vi "QuaternionDecode.vi"(8 "qw":dbl, 9 "qz":dbl, 10 "qy":dbl, 11 "qx":dbl) -> (1 "heading":dbl)   [LabVIEW 2009]
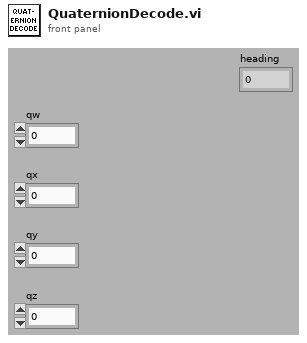
[diagram p1: front panel]
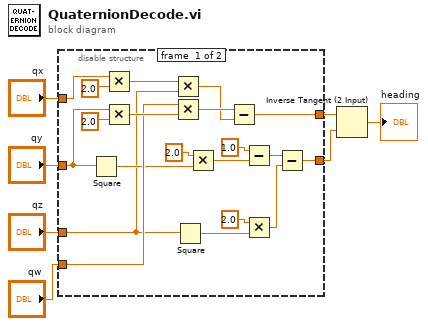
[diagram p0: block diagram]
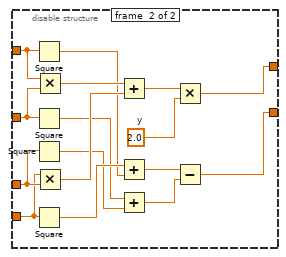
[diagram p2: hidden frame]
diagram:
  n1 = disable-structure shown="Enabled" {
    disable-tunnel: "qw" -> [w25 w36]
    disable-tunnel: "qx" -> [w23 w37]
    disable-tunnel: [w19 w29] -> w5
    disable-tunnel: "qy" -> [w17 w38]
    disable-tunnel: "qz" -> [w13 w39]
    disable-tunnel: [w8 w28] -> w2
    frame #0 {
      n2 = Square(x=w17) -> (x^2=w16:dbl)
      n3 = Multiply(x=w23, y=2.0) -> (x*y=w21:dbl)
      n4 = Multiply(x=w17, y=2.0) -> (x*y=w26:dbl)
      n5 = Multiply(x=w21, y=w13) -> (x*y=w20:dbl)
      n6 = Multiply(x=w25, y=w26) -> (x*y=w24:dbl)
      n7 = Square(x=w13) -> (x^2=w12:dbl)
      n8 = Multiply(x=2.0, y=w16) -> (x*y=w14:dbl)
      n9 = Subtract(x=w24, y=w20) -> (x-y=w19:dbl)
      n10 = Subtract(x=1.0, y=w14) -> (x-y=w10:dbl)
      n11 = Multiply(x=2.0, y=w12) -> (x*y=w9:dbl)
      n12 = Subtract(x=w10, y=w9) -> (x-y=w8:dbl)
    }
    frame #1 {
      w40 = 2.0  # y
      n13 = Square(x=w37) -> (x^2=w31:dbl)
      n14 = Square(x=w38) -> (x^2=w34:dbl)
      n15 = Square(x=w39) -> (x^2=w30:dbl)
      n16 = Square(x=w36) -> (x^2=w35:dbl)
      n17 = Multiply(x=w37, y=w38) -> (x*y=w43:dbl)
      n18 = Multiply(x=w36, y=w39) -> (x*y=w42:dbl)
      n19 = Add(x=w43, y=w42) -> (x+y=w41:dbl)
      n20 = Add(x=w35, y=w31) -> (x+y=w32:dbl)
      n21 = Add(x=w34, y=w30) -> (x+y=w33:dbl)
      n22 = Multiply(x=w41, y=w40) -> (x*y=w29:dbl)
      n23 = Subtract(x=w32, y=w33) -> (x-y=w28:dbl)
    }
  }
  n24 = Inverse Tangent (2 Input)(1:w2, 2:w5) -> (0:→"heading":dbl)
